vi "Process Test Limits.vi"(0 "Signal In":sgl[](array[numeric]), 1 "RMS":dbl[](array[numeric]), 2 "Pk-Pk":dbl[](array[numeric]), 3 "Frequency":dbl[](array[numeric]), 4 "Peaks":dbl[](array[numeric]), 5 "Valleys":dbl[](array[numeric]), 6 "Test Limits":T3, 7 "Sensors":T2(array[cluster]), 9 "Channel":T1) -> (14 "Data Array":string[](array[string]), 16 "Channel Labels":string[](array[string]))   [LabVIEW 2019]
uses:
  Type Defs and Controls/Test Limits.ctl
  Type Defs and Controls/Channel Config.ctl
  <vilib>/Analysis/baseanly.llb/Mean (DBL).vi
  <vilib>/Analysis/NI_AALBase.lvlib
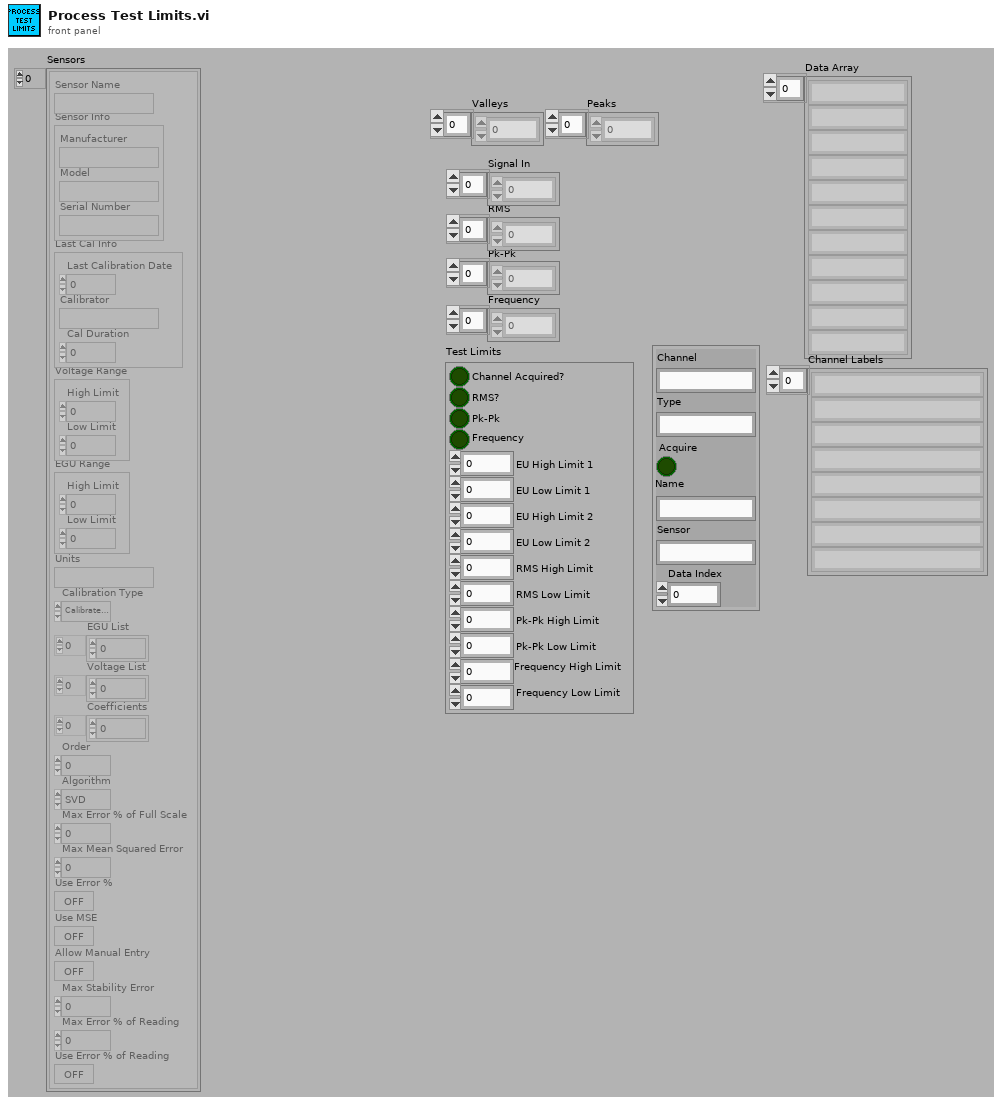
[diagram p1: front panel]
types:
  T1 = typedef "Channel Config.ctl" = cluster{"Channel":string, "Type":string, "Acquire":bool, "Name":string, "Sensor":string, "Data Index":u32}
  T2 = cluster{"Sensor Name":string, "Sensor Info":cluster{"Manufacturer":string, "Model":string, "Serial Number":string}, "Last Cal Info":cluster{"Last Calibration Date":dbl, "Calibrator":string, "Cal Duration":i32}, "Voltage Range":cluster{"High Limit":dbl, "Low Limit":dbl}, "EGU Range":cluster{"High Limit":dbl, "Low Limit":dbl}, "Units":string, "Calibration Type":enum16{"Calibrate Analog", "Compare Analog Calibration"}, "EGU List":dbl[], "Voltage List":dbl[], "Coefficients":dbl[], "Order":i32, "Algorithm":enum32{"SVD", "Givens", "Givens2", "Householder", "LU Decomposition", "Cholesky"}, "Max Error % of Full Scale":dbl, "Max Mean Squared Error":dbl, "Use Error %":bool, "Use MSE":bool, "Allow Manual Entry":bool, "Max Stability Error":dbl, "Max Error % of Reading":dbl, "Use Error % of Reading":bool}[]
  T3 = typedef "Test Limits.ctl" = cluster{"Channel Acquired?":bool, "RMS?":bool, "Pk-Pk":bool, "Frequency":bool, "EU High Limit 1":dbl, "EU Low Limit 1":dbl, "EU High Limit 2":dbl, "EU Low Limit 2":dbl, "RMS High Limit":dbl, "RMS Low Limit":dbl, "Pk-Pk High Limit ":dbl, "Pk-Pk Low Limit":dbl, "Frequency High Limit":dbl, "Frequency Low Limit":dbl}
  T4 = cluster{"Sensor Name":string, "Sensor Info":cluster{"Manufacturer":string, "Model":string, "Serial Number":string}, "Last Cal Info":cluster{"Last Calibration Date":dbl, "Calibrator":string, "Cal Duration":i32}, "Voltage Range":cluster{"High Limit":dbl, "Low Limit":dbl}, "EGU Range":cluster{"High Limit":dbl, "Low Limit":dbl}, "Units":string, "Calibration Type":enum16{"Calibrate Analog", "Compare Analog Calibration"}, "EGU List":dbl[], "Voltage List":dbl[], "Coefficients":dbl[], "Order":i32, "Algorithm":enum32{"SVD", "Givens", "Givens2", "Householder", "LU Decomposition", "Cholesky"}, "Max Error % of Full Scale":dbl, "Max Mean Squared Error":dbl, "Use Error %":bool, "Use MSE":bool, "Allow Manual Entry":bool, "Max Stability Error":dbl, "Max Error % of Reading":dbl, "Use Error % of Reading":bool}
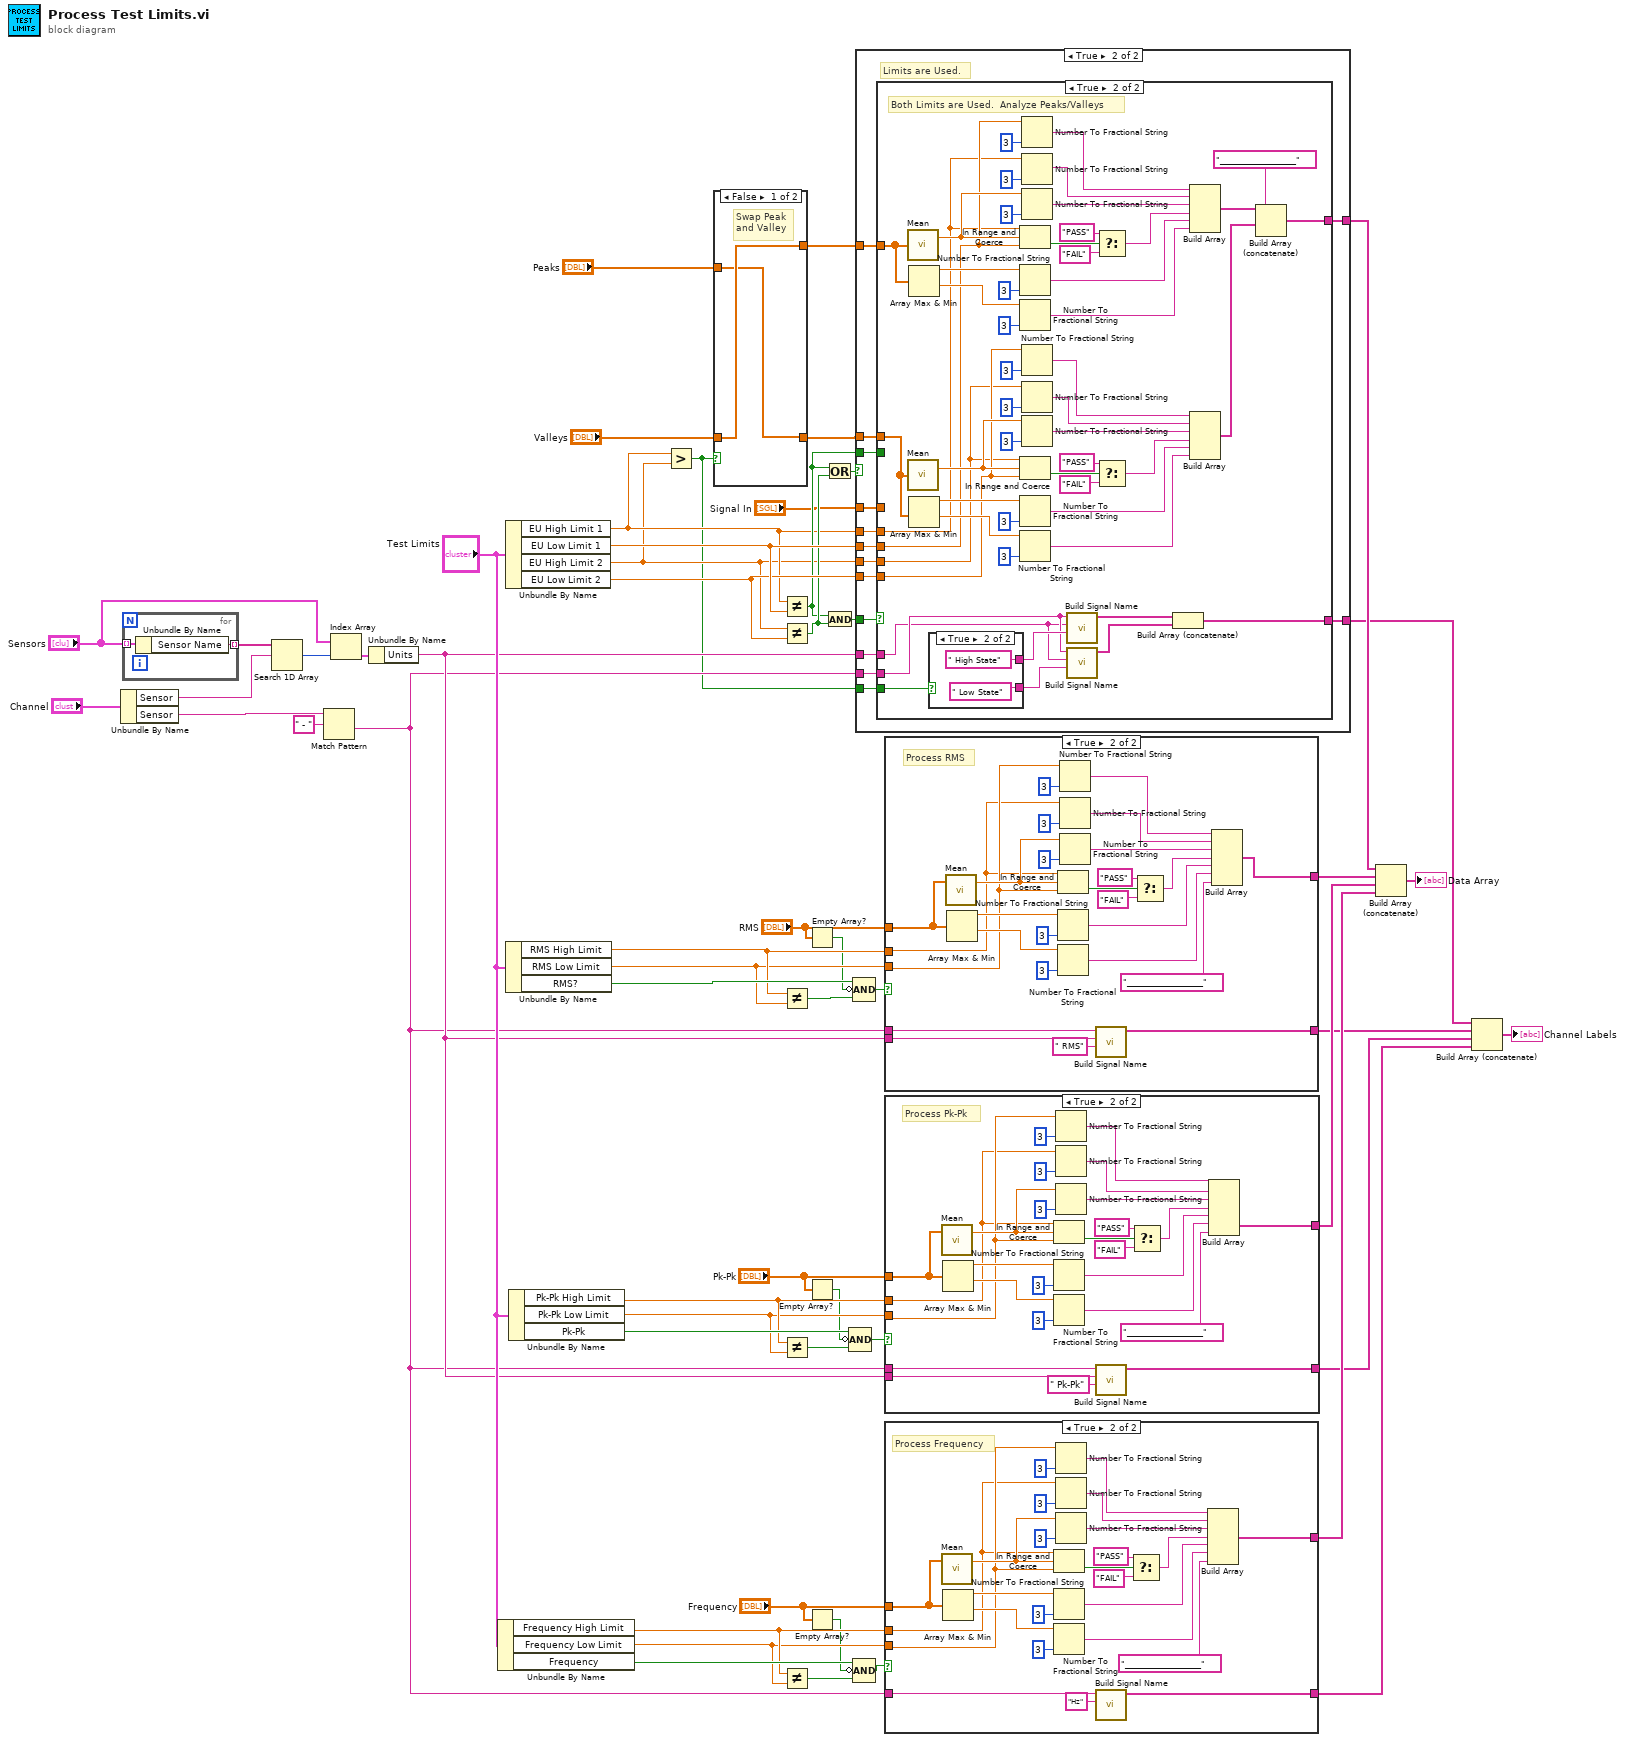
[diagram p0: block diagram]
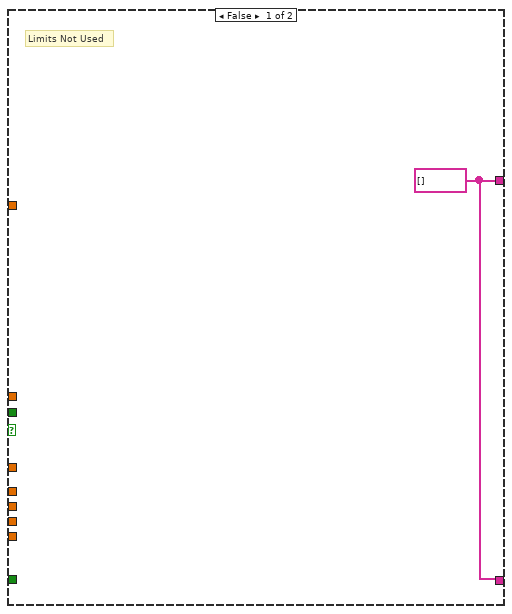
[diagram p3: hidden frame]
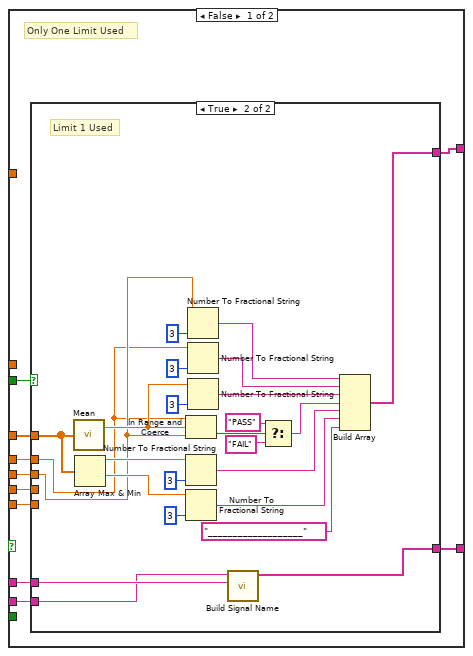
[diagram p4: hidden frame]
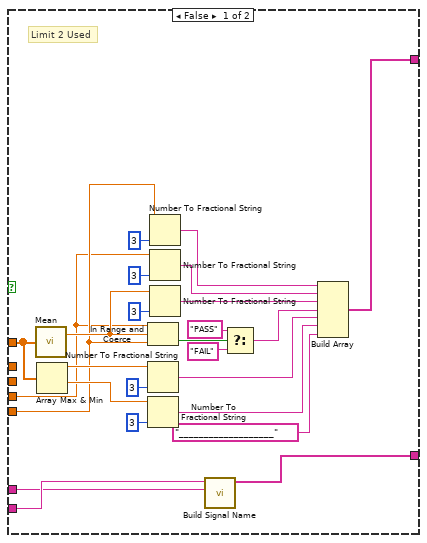
[diagram p5: hidden frame]
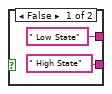
[diagram p6: hidden frame]
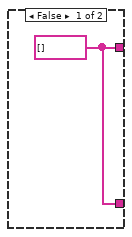
[diagram p7: hidden frame]
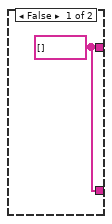
[diagram p8: hidden frame]
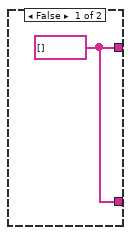
[diagram p9: hidden frame]
diagram:
  n1 = Unbundle By Name("Channel") -> ("Sensor"=w19:string, "Sensor"=w12:string)
  n2 = for {
    tunnel: "Sensors" -> [w58] mode=indexing
    tunnel: [w57] -> w24 mode=indexing
    n3 = Unbundle By Name(w58) -> ("Sensor Name"=w57:string)
  }
  n4 = Search 1D Array(1D array=w24, element=w19) -> (index of element=w23:i32)  [unwired: 1 in]
  n5 = Match Pattern(string=w12, regular expression=" - ") -> (after substring=w10:string)  [unwired: 1 in, 3 out]
  n6 = Index Array(array="Sensors", index=w23) -> (element=w21:T4)
  n7 = Unbundle By Name(w21) -> ("Units"=w16:string)
  n8 = Unbundle By Name("Test Limits") -> ("Frequency High Limit"=w40:dbl, "Frequency Low Limit"=w39:dbl, "Frequency"=w41:bool)
  n9 = Unbundle By Name("Test Limits") -> ("EU High Limit 1"=w9:dbl, "EU Low Limit 1"=w51:dbl, "EU High Limit 2"=w8:dbl, "EU Low Limit 2"=w50:dbl)
  n10 = Unbundle By Name("Test Limits") -> ("RMS High Limit"=w48:dbl, "RMS Low Limit"=w47:dbl, "RMS?"=w49:bool)
  n11 = Unbundle By Name("Test Limits") -> ("Pk-Pk High Limit"=w45:dbl, "Pk-Pk Low Limit"=w44:dbl, "Pk-Pk"=w46:bool)
  n12 = Greater?(x=w9, y=w8) -> (0:w2:bool)
  n13 = case shown="False" w2 {
    tunnel: [w59 w62] -> w5
    tunnel: "Valleys" -> [w60 w62]
    tunnel: "Peaks" -> [w59 w61]
    tunnel: [w60 w61] -> w3
    frame False {
      # "Swap Peak\nand Valley"
    }
    frame True {
    }
  }
  n14 = Not Equal?(x=w9, y=w51) -> (x != y?=w26:bool)
  n15 = Not Equal?(x=w8, y=w50) -> (x != y?=w28:bool)
  n16 = Not Equal?(x=w48, y=w47) -> (x != y?=w38:bool)
  n17 = Not Equal?(x=w45, y=w44) -> (x != y?=w30:bool)
  n18 = Not Equal?(x=w40, y=w39) -> (x != y?=w43:bool)
  n19 = Empty Array?(array="RMS") -> (empty?=w36:bool)
  n20 = Empty Array?(array="Pk-Pk") -> (empty?=w31:bool)
  n21 = Empty Array?(array="Frequency") -> (empty?=w34:bool)
  n22 = Or(x=w26, y=w28) -> (x .or. y?=w27:bool)
  n23 = And(x=w26, y=w28) -> (x .and. y?=w29:bool)
  n24 = Compound Arithmetic op=AND(w46, invert w31, w30) -> (w32:bool)
  n25 = Compound Arithmetic op=AND(w49, invert w36, w38) -> (w33:bool)
  n26 = Compound Arithmetic op=AND(w41, invert w34, w43) -> (w42:bool)
  n27 = case shown="True" w27 {
    tunnel: w9 -> [_ w77]
    tunnel: w51 -> [_ w76]
    tunnel: w8 -> [_ w75]
    tunnel: w50 -> [_ w74]
    tunnel: w3 -> [_ w73]
    tunnel: w5 -> [_ w72]
    tunnel: "Signal In" -> [_ w71]
    tunnel: w29 -> [_ w70]
    tunnel: w26 -> [_ w69]
    tunnel: [w63 w68] -> w25
    tunnel: w16 -> [_ w67]
    tunnel: w10 -> [_ w66]
    tunnel: [w63 w65] -> w18
    tunnel: w2 -> [_ w64]
    frame False {
      w63 = string[] []
      # "Limits Not Used"
    }
    frame True {
      # "Limits are Used."
      n28 = case shown="True" w70 {
        tunnel: w77 -> [w82 w151]
        tunnel: w76 -> [w81 w152]
        tunnel: w75 -> [w85 w155]
        tunnel: w74 -> [w84 w156]
        tunnel: w73 -> [_ w187]
        tunnel: w72 -> [_ w139]
        tunnel: w71 -> [w86 _]
        tunnel: w69 -> [w87 _]
        tunnel: [w83 w160] -> w68
        tunnel: w67 -> [w79 w143]
        tunnel: w66 -> [w80 w145]
        tunnel: [w78 w140] -> w65
        tunnel: w64 -> [_ w138]
        frame False {
          # "Only One Limit Used"
          n29 = case shown="True" w87 {
            tunnel: w86 -> [w101 w126]
            tunnel: w85 -> [w94 _]
            tunnel: w84 -> [w95 _]
            tunnel: [w99 w124] -> w83
            tunnel: w82 -> [_ w119]
            tunnel: w81 -> [_ w120]
            tunnel: w80 -> [w91 w115]
            tunnel: w79 -> [w90 w116]
            tunnel: [w89 w114] -> w78
            frame False {
              # "Limit 2 Used"
              n30 = call-poly <vilib>:"Mean.vi"("X"=w101) -> ("mean"=w100:dbl)  [unwired: 1 out]
              n31 = Array Max & Min(array=w101) -> (max value=w112:sgl, min value=w111:sgl)  [unwired: 2 out]
              n32 = In Range and Coerce(upper limit=w94, x=w100, lower limit=w95) -> (In Range?=w108:bool)  [unwired: 1 out]
              n33 = Number To Fractional String(number=w112, precision (6)=i16 3) -> (F-format string=w103:string)  [unwired: 2 in]
              n34 = Number To Fractional String(number=w111, precision (6)=i16 3) -> (F-format string=w102:string)  [unwired: 2 in]
              n35 = Number To Fractional String(number=w95, precision (6)=i16 3) -> (F-format string=w92:string)  [unwired: 2 in]
              n36 = Number To Fractional String(number=w94, precision (6)=i16 3) -> (F-format string=w93:string)  [unwired: 2 in]
              n37 = Number To Fractional String(number=w100, precision (6)=i16 3) -> (F-format string=w105:string)  [unwired: 2 in]
              n38 = call "Build Signal Name.vi"("Units"=w90, "Signal Name"=w91) -> ("Output"=w89:string[])  [unwired: 9 in]
              n39 = Select(t="PASS" ("format string"), s=w108, f="FAIL" ("format string")) -> (s? t:f=w104:string)
              n40 = Build Array(w92, w93, w105, w104, w103, w102, "___________________" ("format string")) -> (w99:string[])
            }
            frame True {
              # "Limit 1 Used"
              n41 = call-poly <vilib>:"Mean.vi"("X"=w126) -> ("mean"=w125:dbl)  [unwired: 1 out]
              n42 = Array Max & Min(array=w126) -> (max value=w137:sgl, min value=w136:sgl)  [unwired: 2 out]
              n43 = In Range and Coerce(upper limit=w119, x=w125, lower limit=w120) -> (In Range?=w133:bool)  [unwired: 1 out]
              n44 = Number To Fractional String(number=w137, precision (6)=i16 3) -> (F-format string=w128:string)  [unwired: 2 in]
              n45 = Number To Fractional String(number=w136, precision (6)=i16 3) -> (F-format string=w127:string)  [unwired: 2 in]
              n46 = Number To Fractional String(number=w120, precision (6)=i16 3) -> (F-format string=w117:string)  [unwired: 2 in]
              n47 = Number To Fractional String(number=w119, precision (6)=i16 3) -> (F-format string=w118:string)  [unwired: 2 in]
              n48 = Number To Fractional String(number=w125, precision (6)=i16 3) -> (F-format string=w130:string)  [unwired: 2 in]
              n49 = call "Build Signal Name.vi"("Units"=w116, "Signal Name"=w115) -> ("Output"=w114:string[])  [unwired: 9 in]
              n50 = Select(t="PASS" ("format string"), s=w133, f="FAIL" ("format string")) -> (s? t:f=w129:string)
              n51 = Build Array(w117, w118, w130, w129, w128, w127, "___________________" ("format string")) -> (w124:string[])
            }
          }
        }
        frame True {
          w159 = "___________________" ("format string")
          # "Both Limits are Used.  Analyze Peaks/Valleys"
          n52 = call-poly <vilib>:"Mean.vi"("X"=w187) -> ("mean"=w179:dbl)  [unwired: 1 out]
          n53 = call-poly <vilib>:"Mean.vi"("X"=w139) -> ("mean"=w177:dbl)  [unwired: 1 out]
          n54 = Array Max & Min(array=w187) -> (max value=w189:dbl, min value=w188:dbl)  [unwired: 2 out]
          n55 = Array Max & Min(array=w139) -> (max value=w186:dbl, min value=w185:dbl)  [unwired: 2 out]
          n56 = case shown="True" w138 {
            tunnel: [" Low State" ("Units") " High State" ("Units")] -> w146
            tunnel: [" High State" ("Units") " Low State" ("Units")] -> w144
            frame False {
            }
            frame True {
            }
          }
          n57 = In Range and Coerce(upper limit=w151, x=w179, lower limit=w152) -> (In Range?=w176:bool)  [unwired: 1 out]
          n58 = Number To Fractional String(number=w189, precision (6)=i16 3) -> (F-format string=w168:string)  [unwired: 2 in]
          n59 = Number To Fractional String(number=w188, precision (6)=i16 3) -> (F-format string=w167:string)  [unwired: 2 in]
          n60 = In Range and Coerce(upper limit=w155, x=w177, lower limit=w156) -> (In Range?=w171:bool)  [unwired: 1 out]
          n61 = Number To Fractional String(number=w186, precision (6)=i16 3) -> (F-format string=w164:string)  [unwired: 2 in]
          n62 = Number To Fractional String(number=w185, precision (6)=i16 3) -> (F-format string=w163:string)  [unwired: 2 in]
          n63 = Number To Fractional String(number=w152, precision (6)=i16 3) -> (F-format string=w150:string)  [unwired: 2 in]
          n64 = Number To Fractional String(number=w151, precision (6)=i16 3) -> (F-format string=w149:string)  [unwired: 2 in]
          n65 = Number To Fractional String(number=w179, precision (6)=i16 3) -> (F-format string=w170:string)  [unwired: 2 in]
          n66 = Number To Fractional String(number=w156, precision (6)=i16 3) -> (F-format string=w147:string)  [unwired: 2 in]
          n67 = Number To Fractional String(number=w155, precision (6)=i16 3) -> (F-format string=w148:string)  [unwired: 2 in]
          n68 = Number To Fractional String(number=w177, precision (6)=i16 3) -> (F-format string=w166:string)  [unwired: 2 in]
          n69 = call "Build Signal Name.vi"("Added Name"=w146, "Units"=w143, "Signal Name"=w145) -> ("Output"=w142:string[])  [unwired: 8 in]
          n70 = call "Build Signal Name.vi"("Added Name"=w144, "Units"=w143, "Signal Name"=w145) -> ("Output"=w141:string[])  [unwired: 8 in]
          n71 = Select(t="PASS" ("format string"), s=w176, f="FAIL" ("format string")) -> (s? t:f=w169:string)
          n72 = Select(t="PASS" ("format string"), s=w171, f="FAIL" ("format string")) -> (s? t:f=w165:string)
          n73 = Build Array (concatenate)(w142, w141) -> (w140:string[])
          n74 = Build Array(w150, w149, w170, w169, w168, w167) -> (w162:string[])
          n75 = Build Array(w147, w148, w166, w165, w164, w163) -> (w161:string[])
          n76 = Build Array (concatenate)(w162, w159, w161, w159) -> (w160:string[])
        }
      }
    }
  }
  n77 = case shown="True" w33 {
    tunnel: w48 -> [_ w202]
    tunnel: w47 -> [_ w203]
    tunnel: "RMS" -> [_ w207]
    tunnel: [w194 w206] -> w56
    tunnel: w10 -> [_ w199]
    tunnel: w16 -> [_ w198]
    tunnel: [w194 w197] -> w17
    frame False {
      w194 = string[] []
    }
    frame True {
      # "Process RMS"
      n78 = call-poly <vilib>:"Mean.vi"("X"=w207) -> ("mean"=w209:dbl)  [unwired: 1 out]
      n79 = Array Max & Min(array=w207) -> (max value=w220:dbl, min value=w219:dbl)  [unwired: 2 out]
      n80 = In Range and Coerce(upper limit=w202, x=w209, lower limit=w203) -> (In Range?=w216:bool)  [unwired: 1 out]
      n81 = Number To Fractional String(number=w220, precision (6)=i16 3) -> (F-format string=w211:string)  [unwired: 2 in]
      n82 = Number To Fractional String(number=w219, precision (6)=i16 3) -> (F-format string=w210:string)  [unwired: 2 in]
      n83 = Number To Fractional String(number=w203, precision (6)=i16 3) -> (F-format string=w201:string)  [unwired: 2 in]
      n84 = Number To Fractional String(number=w202, precision (6)=i16 3) -> (F-format string=w200:string)  [unwired: 2 in]
      n85 = Number To Fractional String(number=w209, precision (6)=i16 3) -> (F-format string=w213:string)  [unwired: 2 in]
      n86 = call "Build Signal Name.vi"("Added Name"=" RMS", "Units"=w198, "Signal Name"=w199) -> ("Output"=w197:string[])  [unwired: 8 in]
      n87 = Select(t="PASS" ("format string"), s=w216, f="FAIL" ("format string")) -> (s? t:f=w212:string)
      n88 = Build Array(w201, w200, w213, w212, w211, w210, "___________________" ("format string")) -> (w206:string[])
    }
  }
  n89 = case shown="True" w32 {
    tunnel: w45 -> [_ w229]
    tunnel: w44 -> [_ w230]
    tunnel: "Pk-Pk" -> [_ w233]
    tunnel: [w221 w234] -> w55
    tunnel: w10 -> [_ w226]
    tunnel: w16 -> [_ w225]
    tunnel: [w221 w224] -> w15
    frame False {
      w221 = string[] []
    }
    frame True {
      # "Process Pk-Pk"
      n90 = call-poly <vilib>:"Mean.vi"("X"=w233) -> ("mean"=w236:dbl)  [unwired: 1 out]
      n91 = Array Max & Min(array=w233) -> (max value=w247:dbl, min value=w246:dbl)  [unwired: 2 out]
      n92 = In Range and Coerce(upper limit=w229, x=w236, lower limit=w230) -> (In Range?=w243:bool)  [unwired: 1 out]
      n93 = Number To Fractional String(number=w247, precision (6)=i16 3) -> (F-format string=w238:string)  [unwired: 2 in]
      n94 = Number To Fractional String(number=w246, precision (6)=i16 3) -> (F-format string=w237:string)  [unwired: 2 in]
      n95 = Number To Fractional String(number=w230, precision (6)=i16 3) -> (F-format string=w227:string)  [unwired: 2 in]
      n96 = Number To Fractional String(number=w229, precision (6)=i16 3) -> (F-format string=w228:string)  [unwired: 2 in]
      n97 = Number To Fractional String(number=w236, precision (6)=i16 3) -> (F-format string=w240:string)  [unwired: 2 in]
      n98 = call "Build Signal Name.vi"("Added Name"=" Pk-Pk", "Units"=w225, "Signal Name"=w226) -> ("Output"=w224:string[])  [unwired: 8 in]
      n99 = Select(t="PASS" ("format string"), s=w243, f="FAIL" ("format string")) -> (s? t:f=w239:string)
      n100 = Build Array(w227, w228, w240, w239, w238, w237, "___________________" ("format string")) -> (w234:string[])
    }
  }
  n101 = case shown="True" w42 {
    tunnel: w40 -> [_ w255]
    tunnel: w39 -> [_ w256]
    tunnel: "Frequency" -> [_ w260]
    tunnel: [w248 w259] -> w54
    tunnel: w10 -> [_ w252]
    tunnel: [w248 w250] -> w14
    frame False {
      w248 = string[] []
    }
    frame True {
      # "Process Frequency"
      n102 = call-poly <vilib>:"Mean.vi"("X"=w260) -> ("mean"=w272:dbl)  [unwired: 1 out]
      n103 = Array Max & Min(array=w260) -> (max value=w261:dbl, min value=w262:dbl)  [unwired: 2 out]
      n104 = In Range and Coerce(upper limit=w255, x=w272, lower limit=w256) -> (In Range?=w265:bool)  [unwired: 1 out]
      n105 = Number To Fractional String(number=w261, precision (6)=i16 3) -> (F-format string=w270:string)  [unwired: 2 in]
      n106 = Number To Fractional String(number=w262, precision (6)=i16 3) -> (F-format string=w271:string)  [unwired: 2 in]
      n107 = Number To Fractional String(number=w256, precision (6)=i16 3) -> (F-format string=w253:string)  [unwired: 2 in]
      n108 = Number To Fractional String(number=w255, precision (6)=i16 3) -> (F-format string=w254:string)  [unwired: 2 in]
      n109 = Number To Fractional String(number=w272, precision (6)=i16 3) -> (F-format string=w268:string)  [unwired: 2 in]
      n110 = call "Build Signal Name.vi"("Units"="Hz", "Signal Name"=w252) -> ("Output"=w250:string[])  [unwired: 9 in]
      n111 = Select(t="PASS" ("format string"), s=w265, f="FAIL" ("format string")) -> (s? t:f=w269:string)
      n112 = Build Array(w253, w254, w268, w269, w270, w271, "___________________" ("format string")) -> (w259:string[])
    }
  }
  n113 = Build Array (concatenate)(w25, w56, w55, w54) -> (→"Data Array":string[])
  n114 = Build Array (concatenate)(w18, w17, w15, w14) -> (→"Channel Labels":string[])
